vi "Check motion errors.vi"(8 "error in (no error)":errorcluster, 10 "VISA output string":string, 11 "ConfocalStage in":refnum<class "ConfocalStage.lvclass">) -> (0 "error out":errorcluster, 3 "ConfocalStage out":refnum<class "ConfocalStage.lvclass">)   [LabVIEW 2012, in "ConfocalStage.lvclass"]
uses:
  ConfocalStage.lvclass
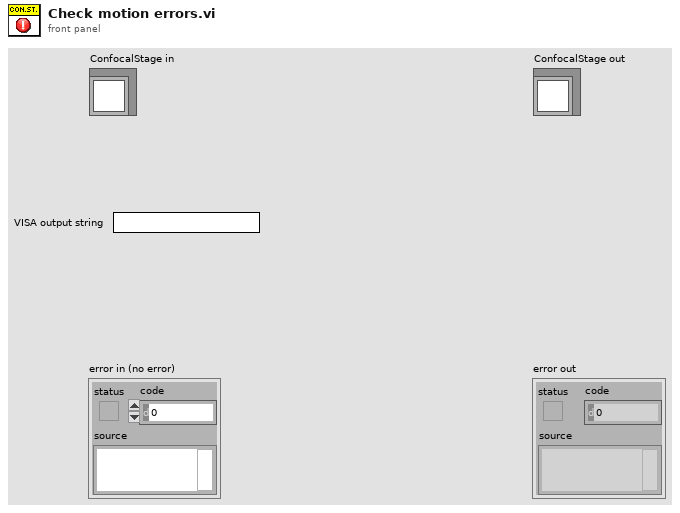
[diagram p1: front panel]
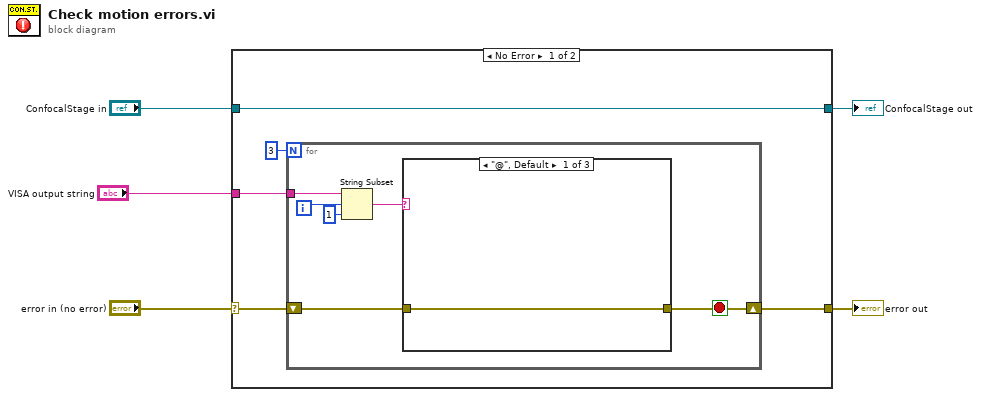
[diagram p0: block diagram]
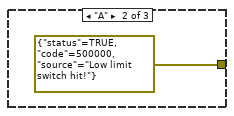
[diagram p2: hidden frame]
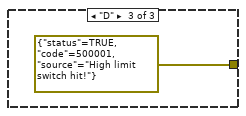
[diagram p3: hidden frame]
diagram:
  n1 = case shown="No Error" "error in (no error)" {
    selector: "error in (no error)" -> [w7 w21]
    tunnel: [w6 w21] -> w4
    tunnel: [w10 w20] -> w2
    tunnel: "ConfocalStage in" -> [w10 w20]
    tunnel: "VISA output string" -> [w8 _]
    frame No Error {
      n2 = for {
        N: 3 -> [_]
        tunnel: w8 -> [w15]
        shift-right: [w11] -> w6
        shift-left: w7 -> [w12]
        i -> [w14]
        stop <- w11 stop-if-true
        n3 = String Subset(string=w15, offset (0)=w14, length (rest)=1 ("length (rest)")) -> (substring=w13:string)
        n4 = case shown="\"@\", Default" w13 {
          tunnel: [w17 errorcluster {"status"=TRUE, "code"=500000, "source"="Low limit switch hit!"} ("error constant") errorcluster {"status"=TRUE, "code"=500001, "source"="High limit switch hit!"} ("error constant")] -> w11
          tunnel: w12 -> [w17 _ _]
          frame "@", Default {
          }
          frame "A" {
          }
          frame "D" {
          }
        }
      }
    }
    frame Error {
    }
  }
  "error out" <- w4
  "ConfocalStage out" <- w2
